vi "SCC_ConnSrv GlobalData.vi"() -> ()   [LabVIEW 2020, in "NI_SCC_ConnSrv.lvlib"]
uses:
  <vilib>/SourceControl/sccconnsrv/NI_SCC_ConnSrv.lvlib
panel:
  in  "ErrorNum Tag":string="<ERRORNUM>"
  in  "SCCserver timeout":i32=10000
  in  "LV_Env_Ref Tag":string="LABVIEW_ENV_REF"
  # "DO NOT LOCALIZE THESE STRINGS!!!!"
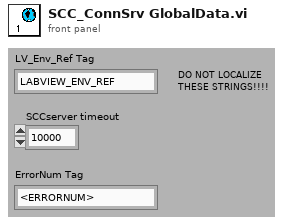
[diagram p1: front panel]
diagram:
